vi "Draw_Calculate Frame Starting Position.vi"(4 "Width":u32, 6 "Height":u32, 8 "Error":errorcluster, 11 "Position":T2) -> (0 "Error Out":errorcluster, 3 "Postion Out":T1)   [LabVIEW 2009]
uses:
  Controls/Enum/RBENUM_Icon Position.ctl
  Controls/Cluster/Cluster_Top Left position.ctl
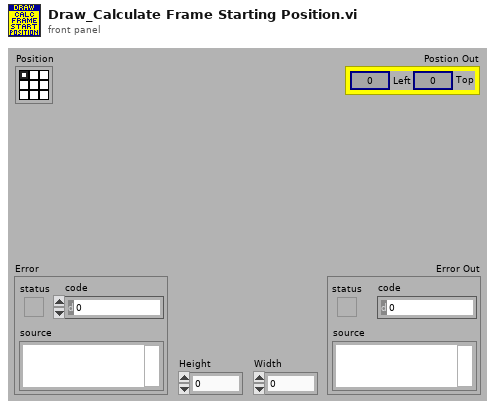
[diagram p1: front panel]
types:
  T1 = typedef "Cluster_Top Left position.ctl" = cluster{"Left":i32, "Top":i32}
  T2 = typedef "RBENUM_Icon Position.ctl" = enum32{"LFT-TOP", "MID-TOP", "RGT-TOP", "LFT-CTR", "MID-CTR", "RGT-CTR", "LFT-BOT", "MID-BOT", "RGT-BOT"}
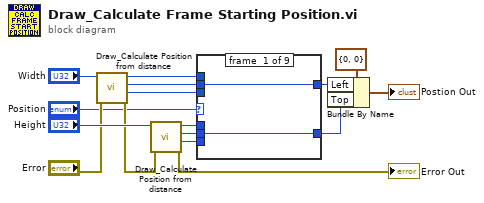
[diagram p0: block diagram]
diagram:
  n1 = call "Draw_Calculate Position from distance.vi"("Error"="Error", "Distance"="Width") -> ("Error Out"=w11:errorcluster, "Far Position Out"=w4:i32, "Center Position Out"=w7:i32, "Near Positoin Out"=w3:i32)  [unwired: 6 in]
  n2 = call "Draw_Calculate Position from distance.vi"("Error"=w11, "Distance"="Height") -> ("Error Out"=→"Error Out":errorcluster, "Far Position Out"=w2:i32, "Center Position Out"=w6:i32, "Near Positoin Out"=w1:i32)  [unwired: 6 in]
  n3 = case shown="\"LFT-CTR\"" "Position" {
    tunnel: w7 -> [w18 _ _ w23 _ w27 _ _ _]
    tunnel: [w18 w19 w21 w23 w25 w27 w29 w31 w34] -> w8
    tunnel: [w17 w20 w22 w24 w26 w28 w30 w32 w33] -> w5
    tunnel: w6 -> [w17 w20 _ _ _ _ _ w32 _]
    tunnel: w4 -> [_ w19 _ _ w25 _ w29 _ _]
    tunnel: w3 -> [_ _ w21 _ _ _ _ w31 w34]
    tunnel: w2 -> [_ _ w22 w24 w26 _ _ _ _]
    tunnel: w1 -> [_ _ _ _ _ w28 w30 _ w33]
    frame #0 {
    }
    frame #1 {
    }
    frame #2 {
    }
    frame #3 {
    }
    frame #4 {
    }
    frame #5 {
    }
    frame #6 {
    }
    frame #7 {
    }
    frame #8 {
    }
  }
  n4 = Bundle By Name(cluster=T1 {"Left"=0, "Top"=0} ("Postion"), "Left"=w8, "Top"=w5) -> (→"Postion Out":T1)
